vi "Get Data.vi"(6 "Samples to Avg":i32, 7 "Cal Files Path":path, 8 "Limits":string[](array[string]), 9 "Available Channels":string[](array[string]), 10 "Channel Config":T1[](array[typedef]), 11 "Netway SNs":i32[](array[numeric])) -> (0 "Error OUT":errorcluster, 2 "Out of Limit?":bool[][](array[boolean]), 3 "Data":string[][](array[string]))   [LabVIEW 2010]
uses:
  Type Defs/DUT and Netway Type Def.ctl
  Type Defs/Netway Ch Strings Cluster Type Def.ctl
  <vilib>/regexp/Match Regular Expression.xnode
  <vilib>/ptbypt/NI_PtbyPt.lvlib
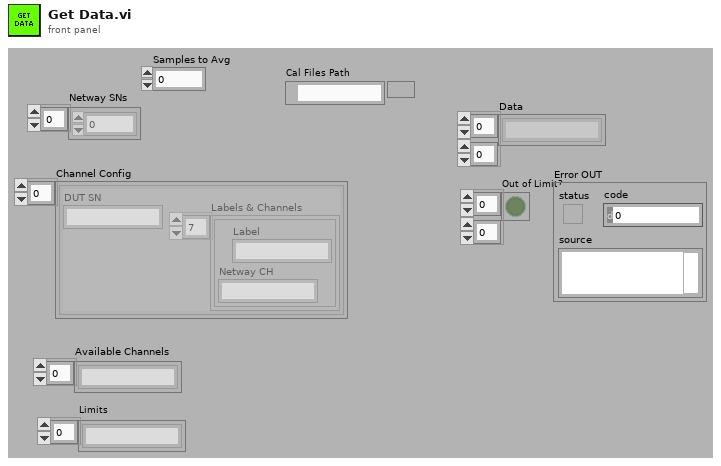
[diagram p1: front panel]
types:
  T1 = typedef "DUT and Netway Type Def.ctl" = cluster{"DUT SN":string, "Labels & Channels":T2[]}
  T2 = typedef "Netway Ch Strings Cluster Type Def.ctl" = cluster{"Label":string, "Netway CH":string}
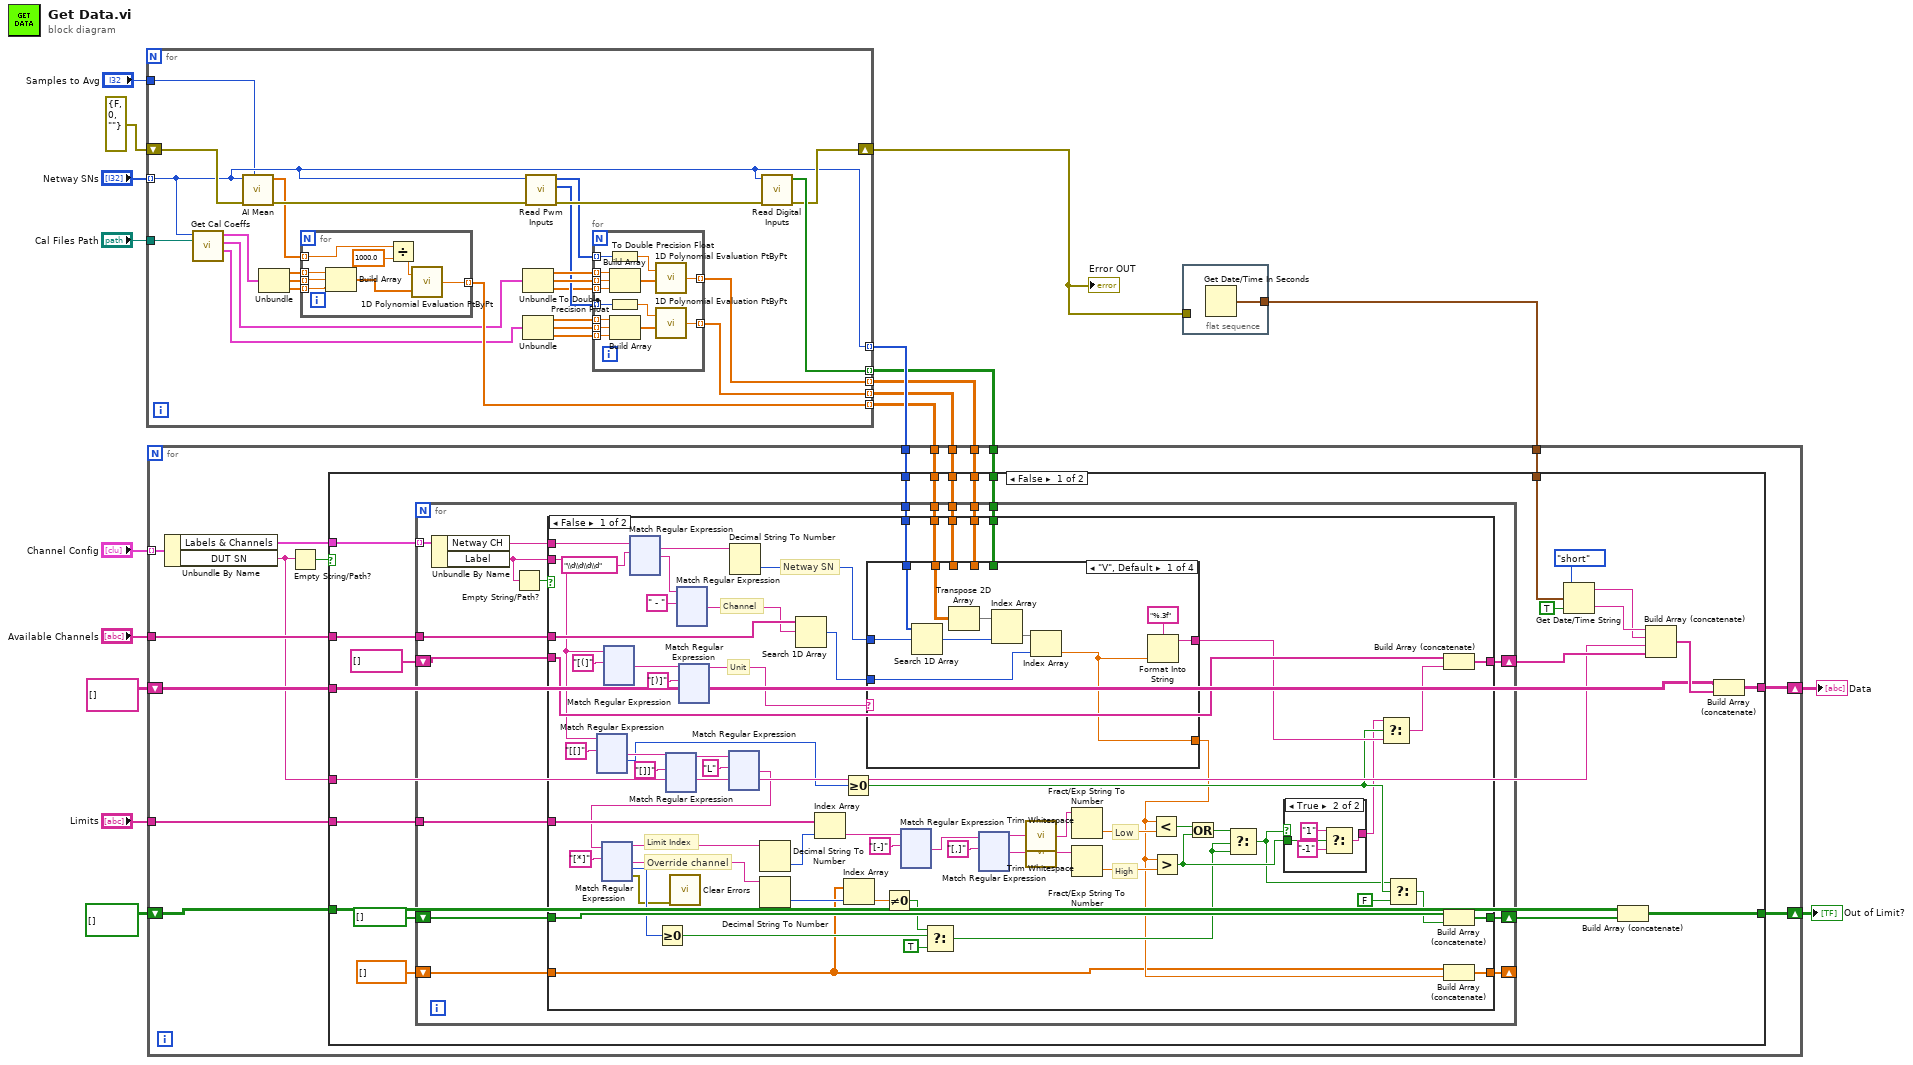
[diagram p0: block diagram]
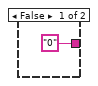
[diagram p2: hidden frame]
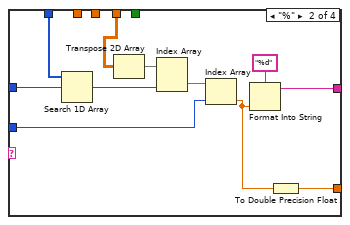
[diagram p3: hidden frame]
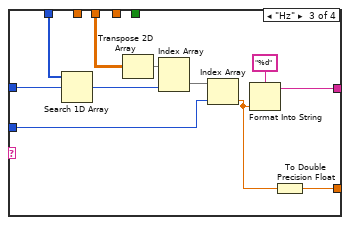
[diagram p4: hidden frame]
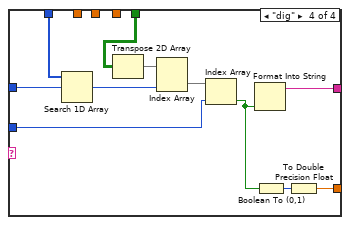
[diagram p5: hidden frame]
diagram:
  n1 = for {
    tunnel: "Netway SNs" -> [w38] mode=indexing
    tunnel: [w42] -> w15 mode=indexing
    tunnel: [w23] -> w14 mode=indexing
    tunnel: [w24] -> w13 mode=indexing
    tunnel: [w34] -> w12 mode=indexing
    tunnel: [w38] -> w16 mode=indexing
    shift-right: [w41] -> w10
    shift-left: errorcluster {"status"=FALSE, "code"=0, "source"=""} ("Error OUT") -> [w40]
    tunnel: "Cal Files Path" -> [w39]
    tunnel: "Samples to Avg" -> [w19]
    n2 = call "Get Cal Coeffs.vi"("Cal Files Path"=w39, "Netway SNs"=w38) -> ("Freq"=w29:cluster{dbl[], dbl[], dbl[]}, "Duty"=w30:cluster{dbl[], dbl[], dbl[]}, "Volts"=w33:cluster{dbl[], dbl[], dbl[]})  [unwired: 7 in]
    n3 = call "AI Mean.vi"("Samples to Avg"=w19, "Error IN"=w40, "Serial Number"=w38) -> ("Error OUT"=w44:errorcluster, "Avg Data"=w37:dbl[])  [unwired: 7 in]
    n4 = Unbundle(w33) -> (w36:dbl[], w35:dbl[], w22:dbl[])
    n5 = for {
      tunnel: w37 -> [w59] mode=indexing
      tunnel: w36 -> [w65] mode=indexing
      tunnel: w35 -> [w64] mode=indexing
      tunnel: [w60] -> w34 mode=indexing
      tunnel: w22 -> [w63] mode=indexing
      n6 = Build Array(w65, w64, w63) -> (w61:dbl[])
      n7 = Divide(x=w59, y=1000.0) -> (x/y=w62:dbl)
      n8 = call <vilib>:"1D Polynomial Evaluation PtByPt.vi"("Coefficients: a"=w61, "x"=w62) -> ("y"=w60:dbl)
    }
    n9 = Unbundle(w30) -> (w32:dbl[], w31:dbl[], w21:dbl[])
    n10 = Unbundle(w29) -> (w28:dbl[], w27:dbl[], w20:dbl[])
    n11 = call <userlib>:"Read Pwm Inputs.vi"("Error IN"=w44, "Serial Number"=w38) -> ("Error OUT"=w43:errorcluster, "Frequency"=w25:i32[], "Duty"=w26:i32[])  [unwired: 7 in]
    n12 = for {
      tunnel: w26 -> [w58] mode=indexing
      tunnel: w32 -> [w55] mode=indexing
      tunnel: w31 -> [w54] mode=indexing
      tunnel: [w46] -> w23 mode=indexing
      tunnel: w28 -> [w52] mode=indexing
      tunnel: w27 -> [w51] mode=indexing
      tunnel: [w45] -> w24 mode=indexing
      tunnel: w25 -> [w57] mode=indexing
      tunnel: w21 -> [w53] mode=indexing
      tunnel: w20 -> [w50] mode=indexing
      n13 = To Double Precision Float(number=w58) -> (double precision float=w56:dbl)
      n14 = Build Array(w55, w54, w53) -> (w49:dbl[])
      n15 = To Double Precision Float(number=w57) -> (double precision float=w48:dbl)
      n16 = Build Array(w52, w51, w50) -> (w47:dbl[])
      n17 = call <vilib>:"1D Polynomial Evaluation PtByPt.vi"("Coefficients: a"=w49, "x"=w56) -> ("y"=w46:dbl)
      n18 = call <vilib>:"1D Polynomial Evaluation PtByPt.vi"("Coefficients: a"=w47, "x"=w48) -> ("y"=w45:dbl)
    }
    n19 = call <userlib>:"Read Digital Inputs.vi"("Error IN"=w43, "Serial Number"=w38) -> ("Error OUT"=w41:errorcluster, "Digital Inputs"=w42:bool[])  [unwired: 8 in]
  }
  "Error OUT" <- w10
  n20 = for {
    tunnel: "Channel Config" -> [w82] mode=indexing
    tunnel: w16 -> [w78]
    tunnel: w15 -> [w74]
    tunnel: w14 -> [w75]
    tunnel: w13 -> [w76]
    tunnel: w12 -> [w80]
    tunnel: "Available Channels" -> [w79]
    tunnel: w9 -> [w77]
    shift-right: [w72] -> w8
    shift-left: string[][] [] -> [w71]
    tunnel: "Limits" -> [w69]
    shift-right: [w68] -> w4
    shift-left: bool[][] [] -> [w67]
    n21 = Unbundle By Name(w82) -> ("Labels & Channels"=w81:T2[], "DUT SN"=w70:string)
    n22 = Empty String/Path?(string/path=w70) -> (empty?=w73:bool)
    n23 = case shown="False" w73 {
      tunnel: w81 -> [w106 _]
      tunnel: w80 -> [w105 _]
      tunnel: w79 -> [w104 _]
      tunnel: w78 -> [w103 _]
      tunnel: w77 -> [w102 _]
      tunnel: w76 -> [w97 _]
      tunnel: w75 -> [w96 _]
      tunnel: w74 -> [w95 _]
      tunnel: [w93 w1352] -> w72
      tunnel: w71 -> [w92 w1352]
      tunnel: w70 -> [w89 _]
      tunnel: w69 -> [w88 _]
      tunnel: [w85 w1351] -> w68
      tunnel: w67 -> [w84 w1351]
      frame False {
        n24 = for {
          tunnel: w106 -> [w123] mode=indexing
          tunnel: w105 -> [w121]
          tunnel: w104 -> [w120]
          tunnel: w103 -> [w119]
          tunnel: w97 -> [w118]
          tunnel: w96 -> [w117]
          tunnel: w95 -> [w116]
          shift-right: [w113] -> w90
          shift-left: string[] [] -> [w112]
          tunnel: w88 -> [w111]
          shift-right: [w110] -> w86
          shift-left: bool[] [] -> [w109]
          shift-right: [w108] -> _
          shift-left: dbl[] [] -> [w107]
          n25 = Unbundle By Name(w123) -> ("Netway CH"=w122:string, "Label"=w115:string)
          n26 = Empty String/Path?(string/path=w115) -> (empty?=w114:bool)
          n27 = case shown="False" w114 {
            tunnel: w122 -> [w183 _]
            tunnel: w115 -> [w166 _]
            tunnel: w121 -> [w182 _]
            tunnel: w120 -> [w180 _]
            tunnel: w119 -> [w178 _]
            tunnel: w118 -> [w176 _]
            tunnel: w117 -> [w175 _]
            tunnel: w116 -> [w174 _]
            tunnel: [w173 w1350] -> w113
            tunnel: w112 -> [w172 w1350]
            tunnel: w111 -> [w165 _]
            tunnel: [w156 w1349] -> w110
            tunnel: w109 -> [w155 w1349]
            tunnel: [w127 w1348] -> w108
            tunnel: w107 -> [w126 w1348]
            frame False {
              # "Limit Index"
              # "Override channel"
              # "High"
              # "Low"
              # "Unit"
              # "Channel"
              # "Netway SN"
              n28 = xnode "Match Regular Expression"("input string"=w166, "regular expression"="[[]") -> ("after match"=w169:string, "offset past match"=w159:i32)  [unwired: 4 in, 3 out]
              n29 = xnode "Match Regular Expression"("input string"=w166, "regular expression"="[(]") -> ("after match"=w184:string)  [unwired: 4 in, 4 out]
              n30 = xnode "Match Regular Expression"("input string"=w183, "regular expression"="\\d\\d\\d\\d") -> ("whole match"=w170:string, "after match"=w187:string)  [unwired: 4 in, 3 out]
              n31 = xnode "Match Regular Expression"("input string"=w169, "regular expression"="[]]") -> ("before match"=w147:string)  [unwired: 4 in, 4 out]
              n32 = xnode "Match Regular Expression"("input string"=w187, "regular expression"=" - ") -> ("after match"=w179:string)  [unwired: 4 in, 4 out]
              n33 = xnode "Match Regular Expression"("input string"=w184, "regular expression"="[)]") -> ("before match"=w181:string)  [unwired: 4 in, 4 out]
              n34 = xnode "Match Regular Expression"("input string"=w147, "regular expression"="L") -> ("after match"=w144:string)  [unwired: 4 in, 4 out]
              n35 = xnode "Match Regular Expression"("input string"=w144, "regular expression"="[*]") -> ("before match"=w143:string, "after match"=w142:string, "offset past match"=w136:i32, "error out"=w132:errorcluster)  [unwired: 4 in, 1 out]
              n36 = Greater Or Equal To 0?(x=w136) -> (x >= 0?=w135:bool)
              n37 = call <vilib>:"Clear Errors.vi"("error in (no error)"=w132) -> ()  [unwired: 6 in, 1 out]
              n38 = Decimal String To Number(string=w170) -> (number=w171:i32)  [unwired: 2 in, 1 out]
              n39 = Decimal String To Number(string=w143) -> (number=w146:i32)  [unwired: 2 in, 1 out]
              n40 = Decimal String To Number(string=w142) -> (number=w141:i32)  [unwired: 2 in, 1 out]
              n41 = Search 1D Array(1D array=w180, element=w179) -> (index of element=w177:i32)  [unwired: 1 in]
              n42 = Index Array(array=w165, index=w146) -> (element=w150:string)
              n43 = Greater Or Equal To 0?(x=w159) -> (x >= 0?=w154:bool)
              n44 = Index Array(array=w126, index=w141) -> (element=w125:dbl)
              n45 = case shown="\"V\", Default" w181 {
                tunnel: [w869 w880 w891 w903] -> w158
                tunnel: w182 -> [w863 _ _ _]
                tunnel: w178 -> [w868 w879 w890 w902]
                tunnel: w171 -> [w867 w878 w889 w901]
                tunnel: w177 -> [w864 w875 w886 w899]
                tunnel: w176 -> [_ _ w884 _]
                tunnel: w175 -> [_ w873 _ _]
                tunnel: w174 -> [_ _ _ w898]
                tunnel: [w861 w871 w882 w894] -> w128
                frame "V", Default {
                  n46 = Search 1D Array(1D array=w868, element=w867) -> (index of element=w866:i32)  [unwired: 1 in]
                  n47 = Transpose 2D Array(2D array=w863) -> (transposed array=w862:dbl[][])
                  n48 = Index Array(array=w862, index (col)=w866) -> (element=w865:dbl[])  [unwired: 1 in]
                  n49 = Index Array(array=w865, index=w864) -> (element=w861:dbl)
                  n50 = Format Into String(format string="%.3f", w861) -> (resulting string=w869:string)  [unwired: 2 in, 1 out]
                }
                frame "%" {
                  n51 = Search 1D Array(1D array=w879, element=w878) -> (index of element=w877:i32)  [unwired: 1 in]
                  n52 = Transpose 2D Array(2D array=w873) -> (transposed array=w874:dbl[][])
                  n53 = Index Array(array=w874, index (col)=w877) -> (element=w876:dbl[])  [unwired: 1 in]
                  n54 = Index Array(array=w876, index=w875) -> (element=w872:dbl)
                  n55 = Format Into String(format string="%d", w872) -> (resulting string=w880:string)  [unwired: 2 in, 1 out]
                  n56 = To Double Precision Float(number=w872) -> (double precision float=w871:dbl)
                }
                frame "Hz" {
                  n57 = Search 1D Array(1D array=w890, element=w889) -> (index of element=w888:i32)  [unwired: 1 in]
                  n58 = Transpose 2D Array(2D array=w884) -> (transposed array=w885:dbl[][])
                  n59 = Index Array(array=w885, index (col)=w888) -> (element=w887:dbl[])  [unwired: 1 in]
                  n60 = Index Array(array=w887, index=w886) -> (element=w883:dbl)
                  n61 = Format Into String(format string="%d", w883) -> (resulting string=w891:string)  [unwired: 2 in, 1 out]
                  n62 = To Double Precision Float(number=w883) -> (double precision float=w882:dbl)
                }
                frame "dig" {
                  n63 = Search 1D Array(1D array=w902, element=w901) -> (index of element=w900:i32)  [unwired: 1 in]
                  n64 = Transpose 2D Array(2D array=w898) -> (transposed array=w897:bool[][])
                  n65 = Index Array(array=w897, index (col)=w900) -> (element=w893:bool[])  [unwired: 1 in]
                  n66 = Index Array(array=w893, index=w899) -> (element=w896:bool)
                  n67 = Format Into String(w896) -> (resulting string=w903:string)  [unwired: 3 in, 1 out]
                  n68 = Boolean To (0,1)(Boolean=w896) -> (0, 1=w895:i16)
                  n69 = To Double Precision Float(number=w895) -> (double precision float=w894:dbl)
                }
              }
              n70 = Not Equal To 0?(x=w125) -> (x != 0?=w124:bool)
              n71 = xnode "Match Regular Expression"("input string"=w150, "regular expression"="[-]") -> ("after match"=w149:string)  [unwired: 4 in, 4 out]
              n72 = Select(t=w124, s=w135, f=TRUE) -> (s? t:f=w129:bool)
              n73 = xnode "Match Regular Expression"("input string"=w149, "regular expression"="[,]") -> ("before match"=w163:string, "after match"=w162:string)  [unwired: 4 in, 3 out]
              n74 = call <vilib>:"Trim Whitespace.vi"("string"=w163) -> ("trimmed string"=w161:string)  [unwired: 1 in]
              n75 = call <vilib>:"Trim Whitespace.vi"("string"=w162) -> ("trimmed string"=w160:string)  [unwired: 1 in]
              n76 = Fract/Exp String To Number(string=w161) -> (number=w140:dbl)  [unwired: 3 in, 1 out]
              n77 = Fract/Exp String To Number(string=w160) -> (number=w139:dbl)  [unwired: 3 in, 1 out]
              n78 = Less?(x=w128, y=w140) -> (x < y?=w138:bool)
              n79 = Greater?(x=w128, y=w139) -> (0:w133:bool)
              n80 = Or(x=w138, y=w133) -> (x .or. y?=w131:bool)
              n81 = Select(t=w131, s=w129, f=w129) -> (s? t:f=w130:bool)
              n82 = case shown="True" w130 {
                tunnel: ["0" ("regular expression") w191] -> w137
                tunnel: w133 -> [_ w192]
                frame False {
                }
                frame True {
                  n83 = Select(t="1" ("regular expression"), s=w192, f="-1" ("regular expression")) -> (s? t:f=w191:string)
                }
              }
              n84 = Select(t=w137, s=w154, f=w158) -> (s? t:f=w157:string)
              n85 = Select(t=w130, s=w154, f=FALSE) -> (s? t:f=w152:bool)
              n86 = Build Array (concatenate)(w172, w157) -> (w173:string[])
              n87 = Build Array (concatenate)(w155, w152) -> (w156:bool[])
              n88 = Build Array (concatenate)(w126, w128) -> (w127:dbl[])
            }
            frame True {
            }
          }
        }
        n89 = Get Date/Time String(date format (0)=enum16{"short", "long", "abbreviated"}."short", seconds (now)=w102, want seconds? (F)=TRUE) -> (date string=w98:string, time string=w99:string)
        n90 = Build Array (concatenate)(w84, w86) -> (w85:bool[][])
        n91 = Build Array (concatenate)(w99, w98, w89, w90) -> (w94:string[])
        n92 = Build Array (concatenate)(w92, w94) -> (w93:string[][])
      }
      frame True {
      }
    }
  }
  "Data" <- w8
  "Out of Limit?" <- w4
  n93 = flat-sequence {
    tunnel: w10 -> [_]
    tunnel: [w1353] -> w9
    frame #0 {
      n94 = Get Date/Time In Seconds() -> (seconds since 1Jan1904=w1353:timestamp)
    }
  }
